vi "Calibrate Varian.vi"(8 "error in":errorcluster, 11 "Sweep Rate":dbl[unit]) -> (0 "error out":errorcluster, 2 "V/T ratio":dbl[unit])   [LabVIEW 2009, in "Varian Magnet.lvclass"]
doc: "This VI is used to calibrate the magnet to get a sense of how quickly it responds to a change in voltage, so we can determine a ratio of V/min to T/min."
uses:
  Varian Magnet.lvclass
  Varian Max Field.vi
panel:
  out "V/min Sweep Rate":dbl[unit]
  out "field rate":dbl[unit]
  out "T2":dbl
  out "T1":dbl
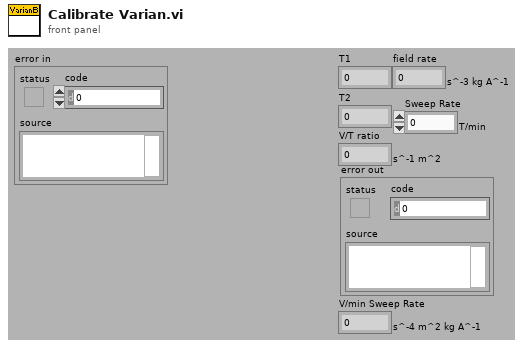
[diagram p1: front panel]
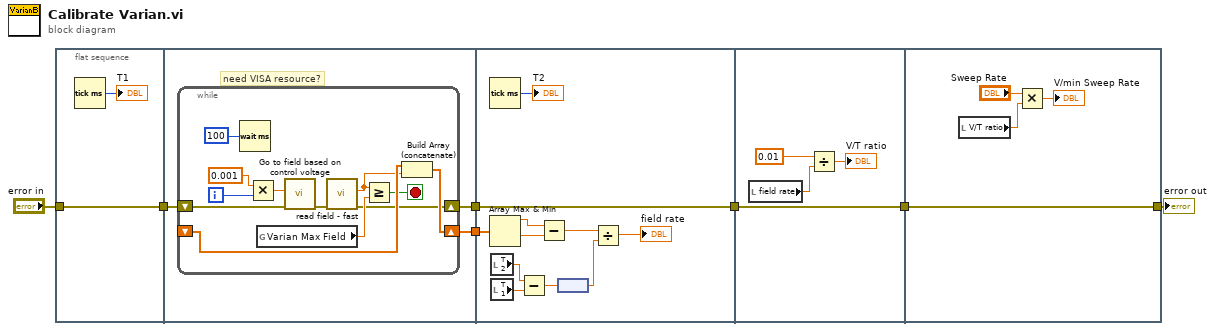
[diagram p0: block diagram]
diagram:
  n1 = flat-sequence {
    tunnel: "error in" -> [w8]
    tunnel: [w8] -> w5
    tunnel: [w12] -> w7
    tunnel: w5 -> [w11]
    tunnel: [w10] -> w4
    tunnel: w7 -> [w34]
    tunnel: w4 -> [w27]
    tunnel: [w27] -> w3
    tunnel: w3 -> [w36]
    tunnel: [w36] -> w1
    tunnel: w1 -> [w43]
    tunnel: [w43] -> w2
    frame #0 {
      n2 = Tick Count (ms)() -> (millisecond timer value=→"T1":u32)
    }
    frame #1 {
      # "need VISA resource?"
      n3 = while {
        shift-right: [w24] -> w12
        shift-left: _ -> [w23]
        shift-right: [w14] -> w10
        shift-left: w11 -> [w13]
        i -> [w18]
        stop <- w19 stop-if-true
        n4 = Wait (ms)(milliseconds to wait=u32 100) -> ()  [unwired: 1 out]
        n5 = Multiply(x=0.001, y=w18) -> (x*y=w16:dbl)
        n6 = global read "Varian Max Field.vi" "Varian Max Field"() -> (w21:dbl[unit])
        n7 = call "Go to field based on control voltage.vi"("error in"=w13, "Control Voltage"=w16) -> ("error out"=w15:errorcluster)  [unwired: 8 in, 1 out]
        n8 = call "read field - fast.vi"("error in (no error)"=w15) -> ("error out"=w14:errorcluster, "Current field (T)"=w20:dbl[unit])  [unwired: 8 in, 1 out]
        n9 = Greater Or Equal?(x=w20, y=w21) -> (x >= y?=w19:bool)
        n10 = Build Array (concatenate)(w23, w20) -> (w24:dbl[unit][])
      }
    }
    frame #2 {
      n11 = Tick Count (ms)() -> (millisecond timer value=→"T2":u32)
      n12 = Array Max & Min(array=w34) -> (max value=w33:dbl[unit], min value=w32:dbl[unit])  [unwired: 2 out]
      n13 = local read "T2"() -> (w31:dbl)
      n14 = local read "T1"() -> (w30:dbl)
      n15 = Subtract(x=w31, y=w30) -> (x-y=w26:dbl)
      n16 = Subtract(x=w33, y=w32) -> (x-y=w29:dbl[unit])
      n17 = node(w26) -> (w25:dbl[unit])
      n18 = Divide(x=w29, y=w25) -> (x/y=→"field rate":dbl[unit])
    }
    frame #3 {
      n19 = local read "field rate"() -> (w38:dbl[unit])
      n20 = Divide(x=dbl[unit] 0.01 ("V/ms"), y=w38) -> (x/y=→"V/T ratio":dbl[unit])
    }
    frame #4 {
      n21 = local read "V/T ratio"() -> (w41:dbl[unit])
      n22 = Multiply(x="Sweep Rate", y=w41) -> (x*y=→"V/min Sweep Rate":dbl[unit])
    }
  }
  "error out" <- w2
